vi "String to Array.vi"() -> ()   [LabVIEW 2011]
panel:
  out "Array":string[](array[string])
  in  "String":string
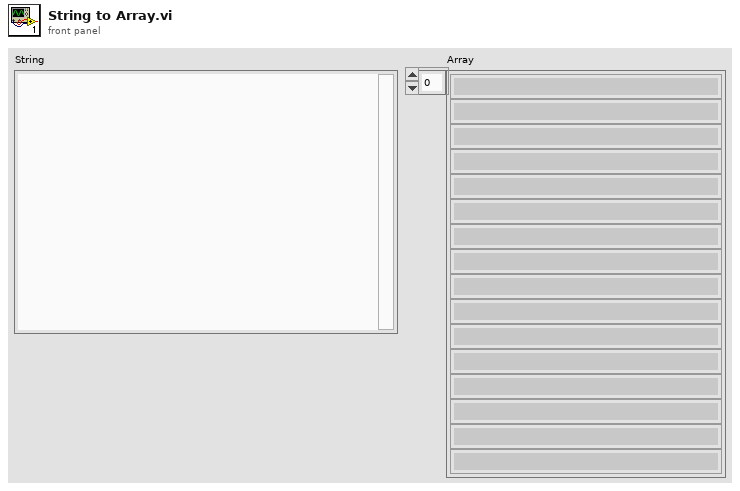
[diagram p1: front panel]
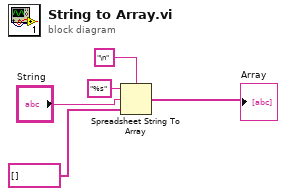
[diagram p0: block diagram]
diagram:
  n1 = Spreadsheet String To Array(delimiter (Tab)="\n", format string="%s", spreadsheet string="String", array type (2D Dbl)=string[] [] ("Array")) -> (array=→"Array":string[])
